vi "MICS Serial Logger.vi"(11 "Array":u8[](array[numeric]) format="%02x") -> ()   [LabVIEW 2020]
panel:
  in  "Clr":bool
  out "Array 2":u8[][](array[numeric]) format="%02x"
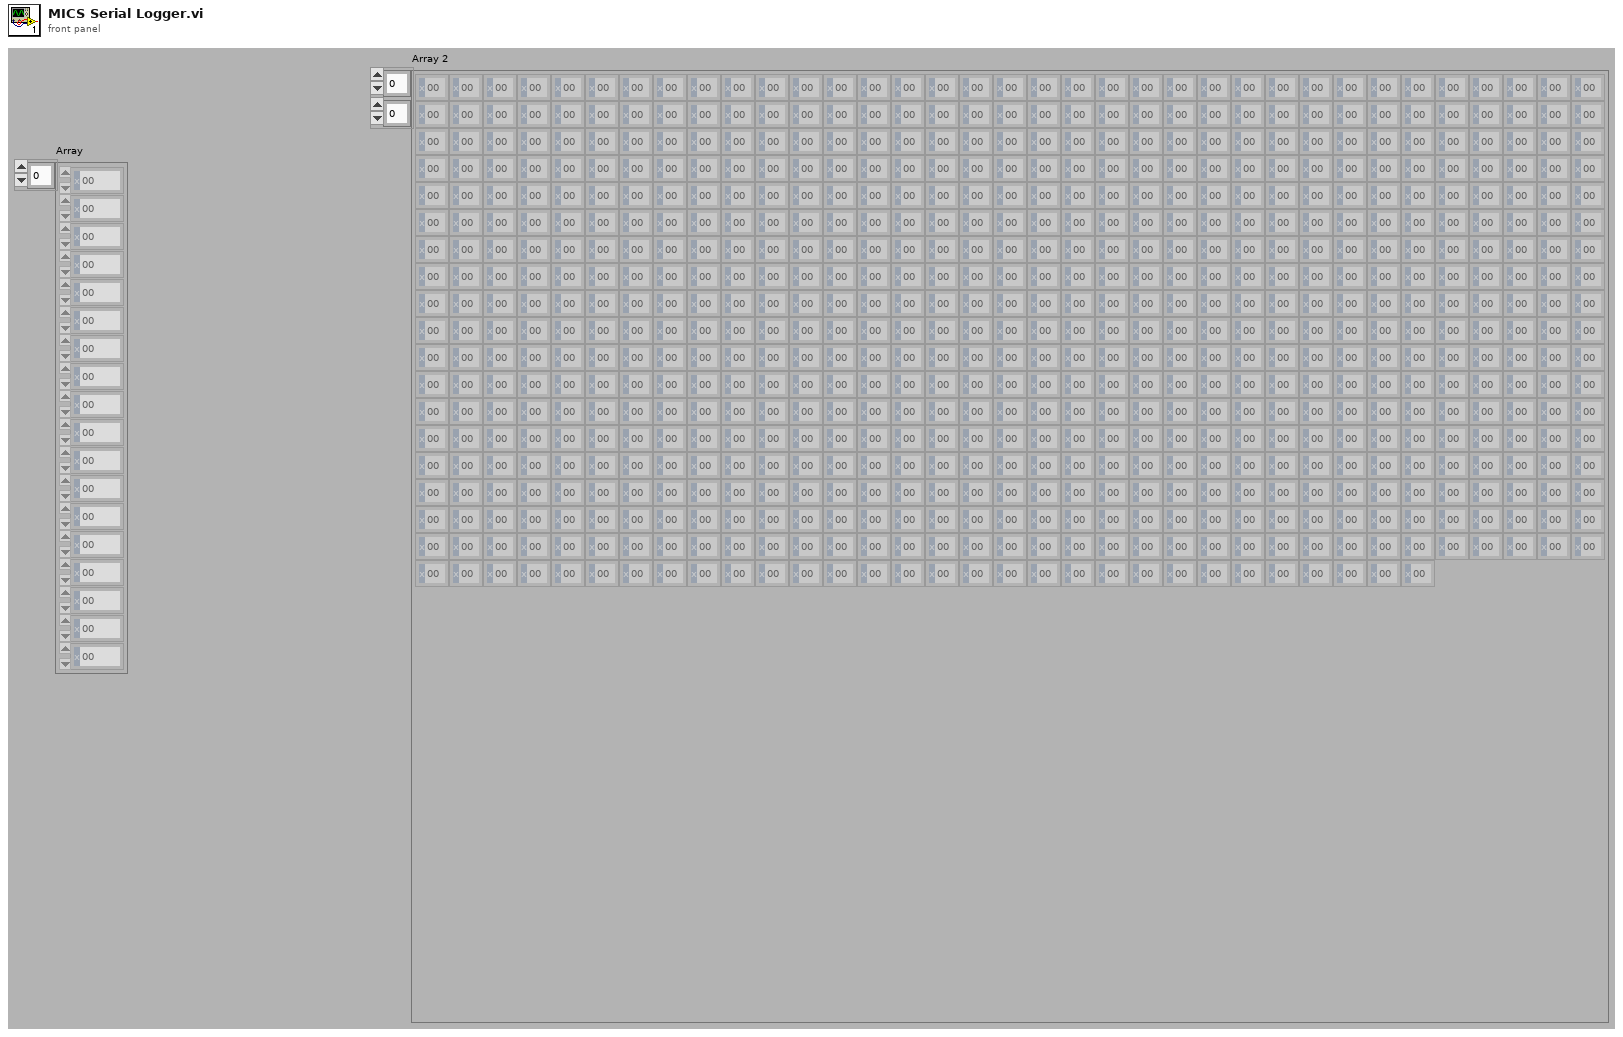
[diagram p1: front panel]
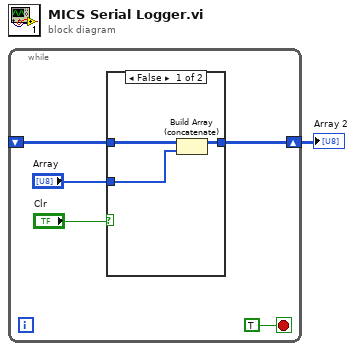
[diagram p0: block diagram]
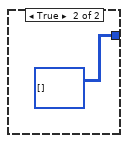
[diagram p2: hidden frame]
diagram:
  n1 = while {
    shift-right: [w5] -> w1
    shift-left: _ -> [w4]
    stop <- TRUE stop-if-true
    n2 = case shown="False" "Clr" {
      tunnel: [w8 u8[][] [] ("Array 2")] -> w5
      tunnel: w4 -> [w9 _]
      tunnel: "Array" -> [w7 _]
      frame False {
        n3 = Build Array (concatenate)(w9, w7) -> (w8:u8[][])
      }
      frame True {
      }
    }
  }
  "Array 2" <- w1
